vi "Tie Game User Prompt and State Transition Out.vi"(8 "error in (no error)":errorcluster) -> (0 "error out":errorcluster, 3 "Next State - Out":T1)   [LabVIEW 2021]
uses:
  Controls/State.ctl
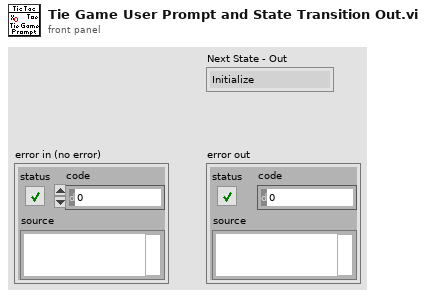
[diagram p1: front panel]
types:
  T1 = typedef "State.ctl" = enum16{"Initialize", "Wait for Event", "Set Left Upp", "Set Left Mid", "Set Left Bot", "Set Middle Upp", "Set Middle Mid", "Set Middle Bot", "Set Right Upp", "Set Right Mid", "Set Right Bot", "Check Game Status", "Exit"}
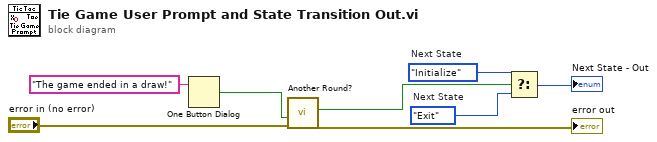
[diagram p0: block diagram]
diagram:
  w7 = State."Initialize"  # Next State
  w8 = State."Exit"  # Next State
  n1 = One Button Dialog(message="The game ended in a draw!") -> (true=w2:bool)  [unwired: 1 in]
  n2 = call "Another Round?"("error in (no error)"="error in (no error)", "Enable"=w2) -> ("error out"=→"error out":errorcluster, "Yes"=w6:bool)  [unwired: 8 in]
  n3 = Select(t=w7, s=w6, f=w8) -> (s? t:f=→"Next State - Out":T1)
